vi "超标留样参数设定.vi"() -> (3 "超标留样":T1={"当前瓶号："=0.0, "平行样："=0.0, "留样瓶数："=0.0, "每瓶次数："=0.0, "每次留样："=0.0, "时间间隔："=0.0, "COD联机："=2, "氨氮联机："=2, "4mA浓度："=0.0, "20mA浓度："=0.0, "超标浓度："=0.0, "4mA浓度："=0.0, "20mA浓度:"=0.0, "超标浓度："=0.0} {"COD联机：" items=["继电器"=1, "模拟输入"=2, "串口连接"=3]; "氨氮联机：" items=["继电器"=1, "模拟输入"=2, "串口连接"=3]})   [LabVIEW 2016, in "德润DR803F超标留样.lvlib"]
uses:
  <vilib>/Utility/miscctls.llb/LVPointTypeDef.ctl
panel:
  out "读取更新":bool
  in  "返回":bool
  in  "当前浓度：":dbl
  in  "超标浓度：":dbl
  in  "20mA浓度：":dbl
  in  "4mA浓度：":dbl
  in  "当前浓度：":dbl
  in  "超标浓度：":dbl
  in  "20mA浓度：":dbl
  in  "4mA浓度：":dbl
  in  "氨氮联机：":u16(ring) items=["继电器"=1, "模拟输入"=2, "串口连接"=3]
  in  "COD联机：":u16(ring) items=["继电器"=1, "模拟输入"=2, "串口连接"=3]
  in  "模拟设置":bool
  in  "每瓶次数：":dbl
  in  "平行样：":dbl
  in  "时间间隔：":dbl
  in  "每次留样：":dbl
  in  "留样瓶数：":dbl
  in  "当前瓶号：":dbl
  # "mg/L"
  # "COD\n模拟\n设置"
  # "mg/L"
  # "mg/L"
  # "mg/L"
  # "mg/L"
  # "氨氮\n模拟\n设置"
  # "mg/L"
  # "mg/L"
  # "mg/L"
  # "在该画面下，可设置该模式下的采样参数，包括当前瓶号、平行样、留样瓶数、每瓶次数、每次留样量和时间间隔（一直超标时的留样时间间隔）。在该画面下，按[]键进入超标选择。"
  # "mL"
  # "min"
  # "1继电器、2模拟输入"
  # "1继电器、2模拟输入"
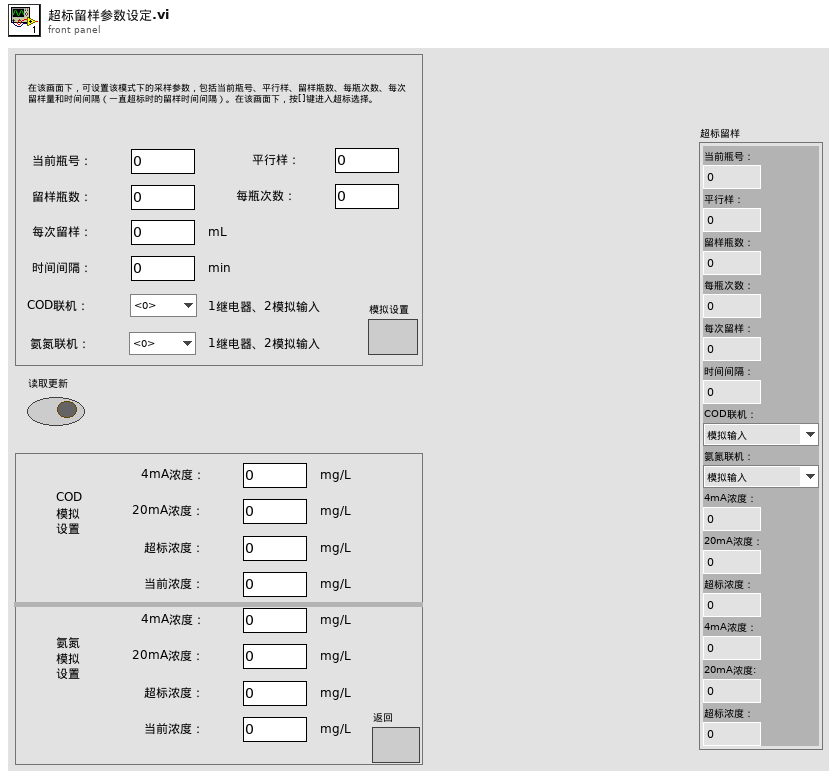
[diagram p1: front panel]
types:
  T1 = cluster{"当前瓶号：":dbl, "平行样：":dbl, "留样瓶数：":dbl, "每瓶次数：":dbl, "每次留样：":dbl, "时间间隔：":dbl, "COD联机：":u16, "氨氮联机：":u16, "4mA浓度：":dbl, "20mA浓度：":dbl, "超标浓度：":dbl, "4mA浓度：":dbl, "20mA浓度:":dbl, "超标浓度：":dbl}
  T2 = typedef "LVPointTypeDef.ctl" = cluster{"Horizontal":i16, "Vertical":i16}
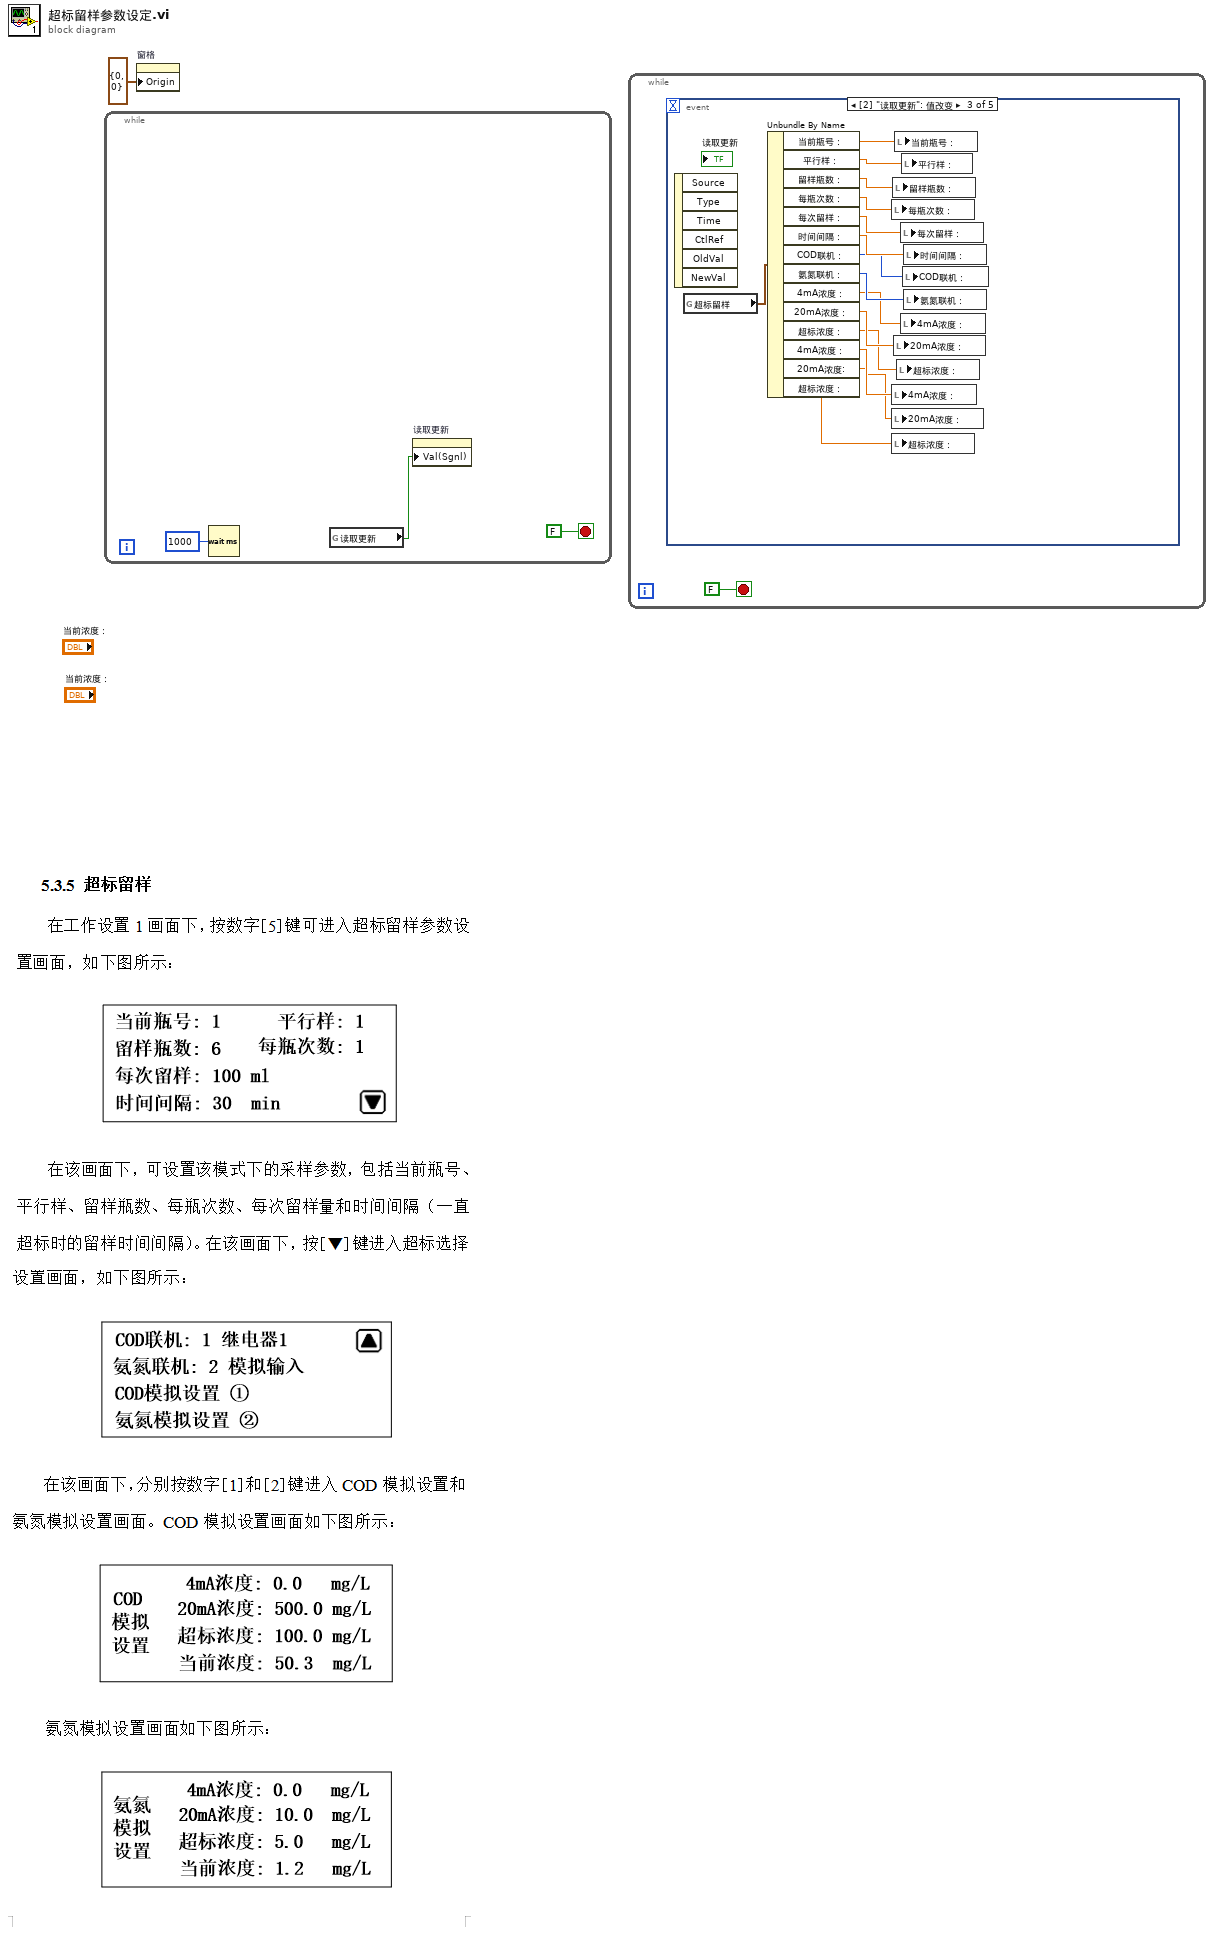
[diagram p0: block diagram]
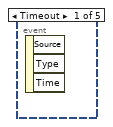
[diagram p2: hidden frame]
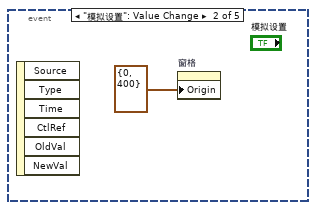
[diagram p3: hidden frame]
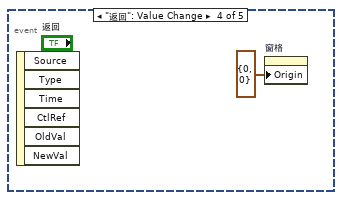
[diagram p4: hidden frame]
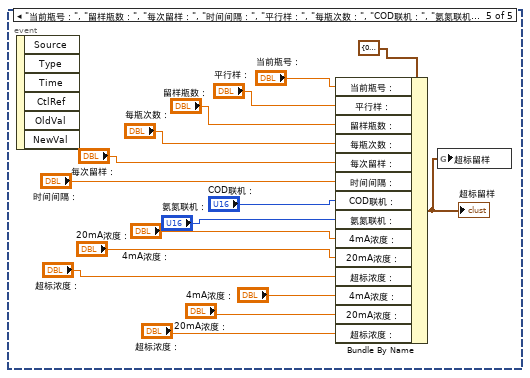
[diagram p5: hidden frame]
diagram:
  n1 = while {
    stop <- FALSE stop-if-true
    n2 = Wait (ms)(milliseconds to wait=u32 1000 ("等待时间（毫秒）")) -> ()  [unwired: 1 out]
    n3 = global read "超标留样全局.vi" "读取更新"() -> (w2:bool)
    n4 = property on="读取更新" class="Bool (严格)"("Val(Sgnl)"=w2) -> ()  [unwired: 2 in, 2 out]
  }
  n5 = property on="窗格" class="Pane"("Origin"=T2 {"Horizontal"=0, "Vertical"=0} ("原点")) -> ()  [unwired: 2 in, 2 out]
  n6 = while {
    stop <- FALSE stop-if-true
    n7 = event shown="[2] \"读取更新\": 值改变" {
      selector: _ -> [_ _ _ _ _]
      dyn-events: _ -> [_ _ _ _ _]
      timeout: _ -> [_ _ _ _ _]
      event Timeout {
        n8 = event-data() -> ()  [unwired: 1 in, 3 out]
      }
      event "模拟设置": Value Change {
        n9 = event-data() -> ()  [unwired: 1 in, 6 out]
        n10 = property on="窗格" class="Pane"("Origin"=T2 {"Horizontal"=0, "Vertical"=400} ("原点")) -> ()  [unwired: 2 in, 2 out]
      }
      event "读取更新": Value Change {
        n11 = event-data() -> ()  [unwired: 1 in, 6 out]
        n12 = global read "超标留样全局.vi" "超标留样"() -> (w21:T1)
        n13 = Unbundle By Name(w21) -> ("当前瓶号："=w20:dbl, "平行样："=w19:dbl, "留样瓶数："=w18:dbl, "每瓶次数："=w17:dbl, "每次留样："=w16:dbl, "时间间隔："=w15:dbl, "COD联机："=w14:u16, "氨氮联机："=w13:u16, "4mA浓度："=w12:dbl, "20mA浓度："=w11:dbl, "超标浓度："=w10:dbl, "4mA浓度："=w9:dbl, "20mA浓度:"=w8:dbl, "超标浓度："=w7:dbl)
        n14 = local write "每瓶次数："(w17) -> ()
        n15 = local write "4mA浓度："(w9) -> ()
        n16 = local write "20mA浓度："(w8) -> ()
        n17 = local write "超标浓度："(w7) -> ()
        n18 = local write "留样瓶数："(w18) -> ()
        n19 = local write "20mA浓度："(w11) -> ()
        n20 = local write "当前瓶号："(w20) -> ()
        n21 = local write "超标浓度："(w10) -> ()
        n22 = local write "每次留样："(w16) -> ()
        n23 = local write "4mA浓度："(w12) -> ()
        n24 = local write "平行样："(w19) -> ()
        n25 = local write "COD联机："(w14) -> ()
        n26 = local write "时间间隔："(w15) -> ()
        n27 = local write "氨氮联机："(w13) -> ()
      }
      event "返回": Value Change {
        n28 = event-data() -> ()  [unwired: 1 in, 6 out]
        n29 = property on="窗格" class="Pane"("Origin"=T2 {"Horizontal"=0, "Vertical"=0} ("原点")) -> ()  [unwired: 2 in, 2 out]
      }
      event "当前瓶号：", "留样瓶数：", "每次留样：", "时间间隔：", "平行样：", "每瓶次数：", "COD联机：", "氨氮联机：", "4mA浓度：", "20mA浓度：", "超标浓度：", "当前浓度：", "4mA浓度：", "20mA浓度：", "超标浓度：", "当前浓度：": Value Change {
        n30 = event-data() -> ()  [unwired: 1 in, 6 out]
        n31 = Bundle By Name(cluster=T1 {"当前瓶号："=0.0, "平行样："=0.0, "留样瓶数："=0.0, "每瓶次数："=0.0, "每次留样："=0.0, "时间间隔："=0.0, "COD联机："=2, "氨氮联机："=2, "4mA浓度："=0.0, "20mA浓度："=0.0, "超标浓度："=0.0, "4mA浓度："=0.0, "20mA浓度:"=0.0, "超标浓度："=0.0} ("超标留样"), "当前瓶号："="当前瓶号：", "平行样："="平行样：", "留样瓶数："="留样瓶数：", "每瓶次数："="每瓶次数：", "每次留样："="每次留样：", "时间间隔："="时间间隔：", "COD联机："="COD联机：", "氨氮联机："="氨氮联机：", "4mA浓度："="4mA浓度：", "20mA浓度："="20mA浓度：", "超标浓度："="超标浓度：", "4mA浓度："="4mA浓度：", "20mA浓度："="20mA浓度：", "超标浓度："="超标浓度：") -> (w38:T1)
        "超标留样" <- w38
        n32 = global write "超标留样全局.vi" "超标留样"(w38) -> ()
      }
    }
  }
